vi "RotateInputVector.vi"(9 "gyro offset":dbl, 10 "y":dbl, 11 "x":dbl) -> (2 "y":dbl, 3 "x":dbl)   [LabVIEW 2013]
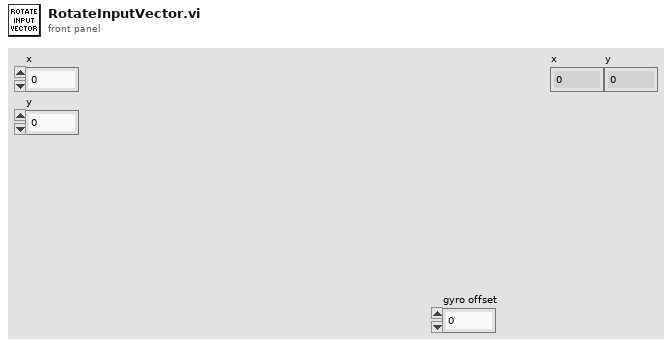
[diagram p1: front panel]
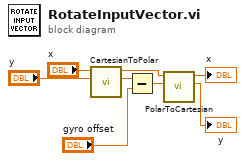
[diagram p0: block diagram]
diagram:
  n1 = call "CartesianToPolar.vi"("y"="y", "x"="x") -> ("theta (radians)"=w7:dbl, "r"=w8:dbl)  [unwired: 8 in]
  n2 = Subtract(x=w7, y="gyro offset") -> (x-y=w6:dbl)
  n3 = call "PolarToCartesian.vi"("theta (radians)"=w6, "r"=w8) -> ("y"=→"y":dbl, "x"=→"x":dbl)  [unwired: 8 in]
